vi "Apply Fade.vi"(0 "Channel in":refnum<class "Channel.lvclass">, 5 "Array in":dbl[](array[numeric]), 7 "Fs (Hz)":dbl, 11 "error in (no error)":errorcluster, 12 "first":bool, 13 "last":bool) -> (4 "Channel out":refnum<class "Channel.lvclass">, 6 "Array out":dbl[](array[numeric]), 15 "error out":errorcluster)   [LabVIEW 2020, in "Channel.lvclass"]
uses:
  Channel.lvclass
  Channel.lvclass/Channel.ctl
  <vilib>/Analysis/NI_AALBase.lvlib
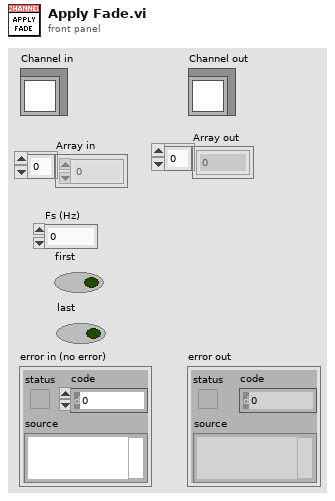
[diagram p1: front panel]
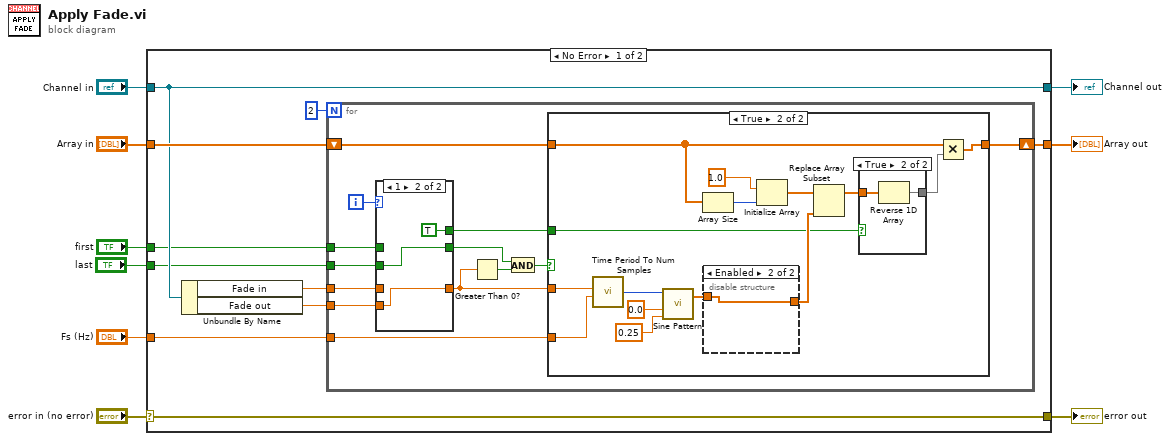
[diagram p0: block diagram]
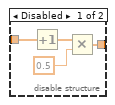
[diagram p3: hidden frame]
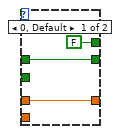
[diagram p5: hidden frame]
diagram:
  n1 = case shown="No Error" "error in (no error)" {
    selector: "error in (no error)" -> [w19 w65]
    tunnel: [w19 w65] -> w8
    tunnel: [w16 w64] -> w6
    tunnel: "Channel in" -> [w16 w64]
    tunnel: "Array in" -> [w18 w63]
    tunnel: [w17 w63] -> w4
    tunnel: "first" -> [w14 _]
    tunnel: "Fs (Hz)" -> [w15 _]
    tunnel: "last" -> [w11 _]
    frame No Error {
      n2 = Unbundle By Name(w16) -> ("Fade in"=w13:dbl, "Fade out"=w12:dbl)
      n3 = for {
        N: 2 -> [_]
        tunnel: w15 -> [w30]
        tunnel: w14 -> [w25]
        tunnel: w13 -> [w29]
        tunnel: w12 -> [w28]
        shift-right: [w31] -> w17
        shift-left: w18 -> [w32]
        tunnel: w11 -> [w27]
        i -> [w26]
        n4 = case shown="1" w26 {
          tunnel: [w58 w61] -> w24
          tunnel: w29 -> [w58 _]
          tunnel: w28 -> [_ w61]
          tunnel: w27 -> [_ w62]
          tunnel: w25 -> [w59 _]
          tunnel: [w59 w62] -> w22
          tunnel: [FALSE TRUE] -> w20
          frame 0, Default {
          }
          frame 1 {
          }
        }
        n5 = Greater Than 0?(x=w24) -> (x > 0?=w23:bool)
        n6 = And(x=w22, y=w23) -> (x .and. y?=w21:bool)
        n7 = case shown="True" w21 {
          tunnel: w32 -> [w33 w43]
          tunnel: [w33 w42] -> w31
          tunnel: w30 -> [_ w41]
          tunnel: w24 -> [_ w40]
          tunnel: w20 -> [_ w34]
          frame False {
          }
          frame True {
            n8 = call "Time Period To Num Samples.vi"("Duration (ms)"=w40, "Sampling rate (Hz)"=w41) -> ("Samples"=w47:i32)  [unwired: 5 in]
            n9 = call <vilib>:"Sine Pattern.vi"("cycles"=0.25, "phase(degrees)"=0.0, "samples"=w47) -> ("Sinusoidal Pattern"=w45:dbl[])  [unwired: 1 in, 1 out]
            n10 = Array Size(array=w43) -> (size(s)=w48:i32)
            n11 = disable-structure shown="Enabled" {
              disable-tunnel: w45 -> [w50 w53]
              disable-tunnel: [w49 w53] -> w37
              frame Disabled {
                n12 = Increment(x=w50) -> (x+1=w52:dbl[])
                n13 = Multiply(x=w52, y=0.5) -> (x*y=w49:dbl[])
              }
              frame Enabled {
              }
            }
            n14 = Initialize Array(1.0 ("element"), w48) -> (w46:dbl[])
            n15 = Replace Array Subset(array=w46, new element=w37) -> (w36:dbl[])  [unwired: 1 in]
            n16 = case shown="True" w34 {
              tunnel: w36 -> [w54 w56]
              tunnel: [w54 w55] -> w35
              frame False {
              }
              frame True {
                n17 = Reverse 1D Array(array=w56) -> (reversed array=w55:dbl[])
              }
            }
            n18 = Multiply(x=w43, y=w35) -> (x*y=w42:dbl[])
          }
        }
      }
    }
    frame Error {
    }
  }
  "error out" <- w8
  "Channel out" <- w6
  "Array out" <- w4
